vi "WFS Take Spotfield Image Auto Expos.vi"(8 "error in (no error)":errorcluster {"code" format="%.0x"}, 11 "instrument handle":refnum<visa-resource-name>) -> (0 "error out":errorcluster {"code" format="%.0x"}, 1 "Master Gain Act":dbl, 2 "Exposure Time Act":dbl, 3 "instrument handle out":refnum<visa-resource-name>)   [LabVIEW 2020]
doc: "This VI tries to find optimal exposure and gain settings and then it receives a spotfield image from the WFS camera into a driver buffer. The reference to this buffer is provided by VI GetSpotfieldImage() and an image copy is returned by VI GetSpotfieldImageCopy().\n\nThe exposure and gain settings used for this image are returned.\n\nIn case of still unsuited image exposure the VI sets the appropriate status bits. Use VI GetStatus() to check the reason.\n\nBit Name Meaning if bit is set\n\n0x00000002 WFS_STATBIT_PTH (2) Power Too High (cam saturated)\n0x00000004 WFS_STATBIT_PTL (4) Power Too Low (low cam digits)\n0x00000008 WFS_STATBIT_HAL (8) High Ambient Light\n\nYou may repeate calling the VI until these status bits are cleared.\n\n\nWhen the trigger capability is activated by VI SetTriggerMode() this VI will wait for a trigger event for a short period of time (WFS_TIMEOUT_CAPTURE_TRIGGER (0.1) = 0.1 sec.) prior to start exposure and will return with error WFS_ERROR_AWAITING_TRIGGER (-1074001642) if no trigger event occured.\nYou need to repeate calling this VI until this error and status bit WFS_STATBIT_ATR (128) disappear.\n\nNote: This VI is not available in Highspeed Mode!"
uses:
  WFS_32.dll
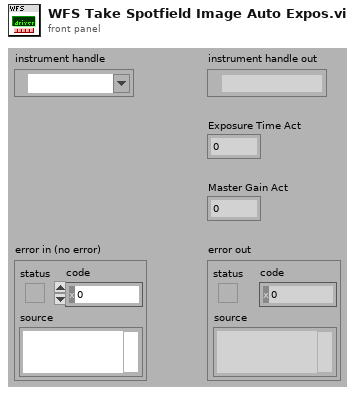
[diagram p1: front panel]
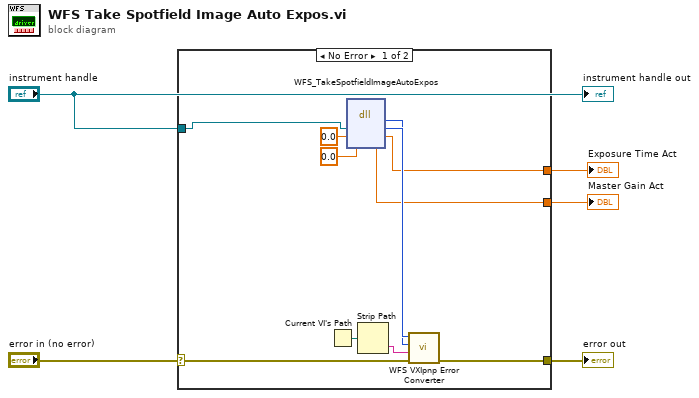
[diagram p0: block diagram]
diagram:
  n1 = case shown="No Error" "error in (no error)" {
    selector: "error in (no error)" -> [w11 w17]
    tunnel: [w10 w17] -> w5
    tunnel: "instrument handle" -> [w15 _]
    tunnel: [w8 _] -> w2
    tunnel: [w6 _] -> w1
    frame No Error {
      n2 = Current VI's Path() -> (path=w16:path)
      n3 = dll-call lib="WFS_*.*" fn="WFS_TakeSpotfieldImageAutoExpos"("Instrument Handle"=w15, "Exposure Time Act"=0.0, "Master Gain Act"=0.0) -> (w13:i32, "Instrument Handle"=w14:u32, "Exposure Time Act"=w8:dbl, "Master Gain Act"=w6:dbl)  [unwired: 3 in, 2 out]
      n4 = Strip Path(path=w16) -> (name=w12:string)  [unwired: 1 out]
      n5 = call "WFS VXIpnp Error Converter.vi"("error in (no error)"=w11, "Name Of VI (\"\")"=w12, "CVI Error Code (0)"=w13, "instrument handle"=w14) -> ("error out"=w10:errorcluster)  [unwired: 6 in, 1 out]
    }
    frame Error {
    }
  }
  "error out" <- w5
  "Exposure Time Act" <- w2
  "Master Gain Act" <- w1
  "instrument handle out" <- "instrument handle"
